vi "DeleteFolders.vi"(8 "error in (no error)":errorcluster, 11 "path":path) -> (0 "error out":errorcluster)   [LabVIEW 2017]
uses:
  <vilib>/Utility/sysdir.llb/System Directory Type.ctl
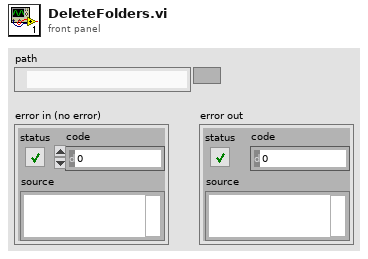
[diagram p1: front panel]
types:
  T1 = typedef "System Directory Type.ctl" = i32
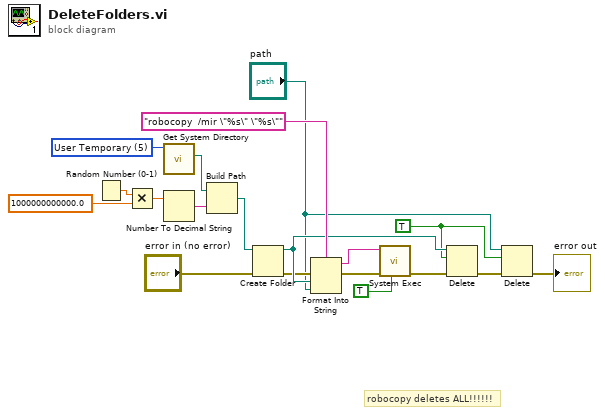
[diagram p0: block diagram]
diagram:
  w3 = TRUE ("entire hierarchy (F)")
  w19 = T1 5 items=["User Home"=0, "User Desktop"=1, "User Documents"=2, "User Application Data"=3, "User Preferences"=4, "User Temporary"=5, "Public Documents"=6, "Public Application Data"=7, "Public Preferences"=8, "Public Cache"=13, "System Core Libraries"=9, "System Installed Libraries"=10, "Application Files"=11, "Boot Volume Root"=12] ("system directory type")
  # "robocopy deletes ALL!!!!!!"
  n1 = Random Number (0-1)() -> (number: 0 to 1=w17:dbl)
  n2 = Multiply(x=w17, y=1000000000000.0) -> (x*y=w15:dbl)
  n3 = call <vilib>:"Get System Directory.vi"("system directory type"=w19) -> ("system directory"=w18:path)  [unwired: 10 in]
  n4 = Number To Decimal String(number=w15) -> (decimal integer string=w14:string)  [unwired: 1 in]
  n5 = Build Path(base path=w18, name or relative path=w14) -> (appended path=w13:path)
  n6 = Create Folder(path (use dialog)=w13, error in="error in (no error)") -> (created path=w11:path, error out=w8:errorcluster)  [unwired: 1 in, 1 out]
  n7 = Format Into String(format string="robocopy  /mir \"%s\" \"%s\"", error in=w8, w11, "path") -> (resulting string=w10:string, error out=w9:errorcluster)  [unwired: 1 in]
  n8 = call <vilib>:"System Exec.vi"("run minimized? (F)"=TRUE, "error in (no error)"=w9, "command line"=w10) -> ("error out"=w6:errorcluster)  [unwired: 5 in, 3 out]
  n9 = Delete(path (use dialog)=w11, entire hierarchy (F)=w3, error in=w6) -> (error out=w5:errorcluster)  [unwired: 2 in, 2 out]
  n10 = Delete(path (use dialog)="path", entire hierarchy (F)=w3, error in=w5) -> (error out=→"error out":errorcluster)  [unwired: 2 in, 2 out]
